vi "Display Info.vi"(7 "Layout ref":refnum<vi>, 8 "error in (no error)":errorcluster, 9 "Modify (F) /Add [T]":bool=TRUE, 10 "Names in use":string[](array[string])=["PB"], 11 "SRS_DS345 in":refnum<class "SRS_DS345.lvclass">=refnum) -> (0 "error out":errorcluster, 1 "Names in use out":string[](array[string]), 2 "Changes Made?":bool, 3 "SRS_DS345 out":refnum<class "SRS_DS345.lvclass">)   [LabVIEW 2013, in "SRS_DS345.lvclass"]
uses:
  SRS_DS345.lvclass
  ColumnVIs/SingleValCol/SingleValCol.lvclass
  TypeDefs/ColumnAppearCluster.ctl
  SRS_DS345.lvclass/SRS_DS345.ctl
  ColumnVIs/Column/Column.lvclass
panel:
  in  "Function Type Column Appearance":T1={"Column Name"="Func Type", "Width"=30, "Bkgd"=[16448250], "Text"=[0]}
  in  "Offset Column Appearance":T1={"Column Name"="Offset", "Width"=30, "Bkgd"=[16448250], "Text"=[0]}
  in  "Amplitude Column Apperance":T1={"Column Name"="Amplitude", "Width"=30, "Bkgd"=[16448250], "Text"=[0]}
  in  "Freq Column Appearance":T1={"Column Name"="Frequency", "Width"=30, "Bkgd"=[16448250], "Text"=[0]}
  in  "Cancel":bool
  in  "Done":bool
  in  "Hardware Settings":T2={"PB Trigger Line"=65535, "Serial Port"=""}
  in  "Device Description":string
  in  "Name":string
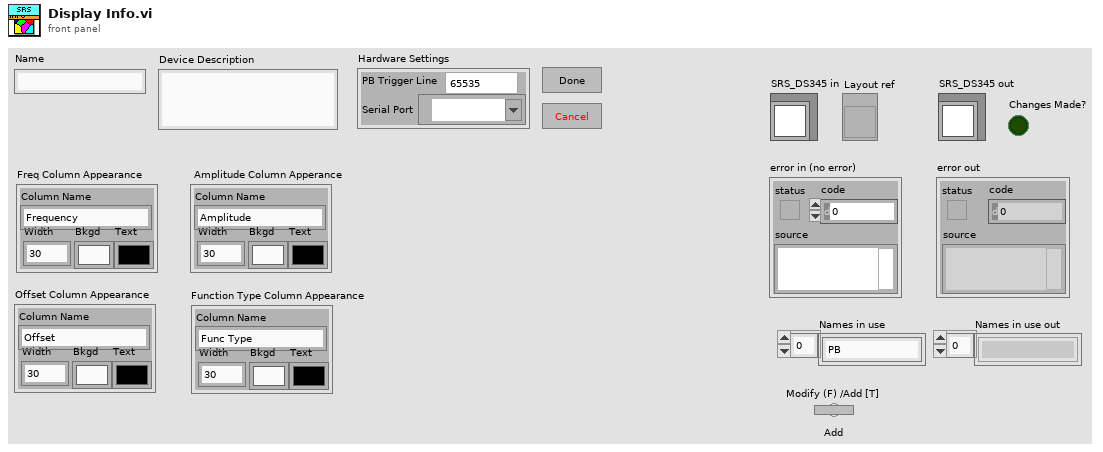
[diagram p1: front panel]
types:
  T1 = typedef "ColumnAppearCluster.ctl" = cluster{"Column Name":string, "Width":u32, "Bkgd":u32[], "Text":u32[]}
  T2 = cluster{"PB Trigger Line":u16, "Serial Port":refnum<visa-resource-name>}
  T3 = cluster{u16, "Serial Port":refnum<visa-resource-name>}
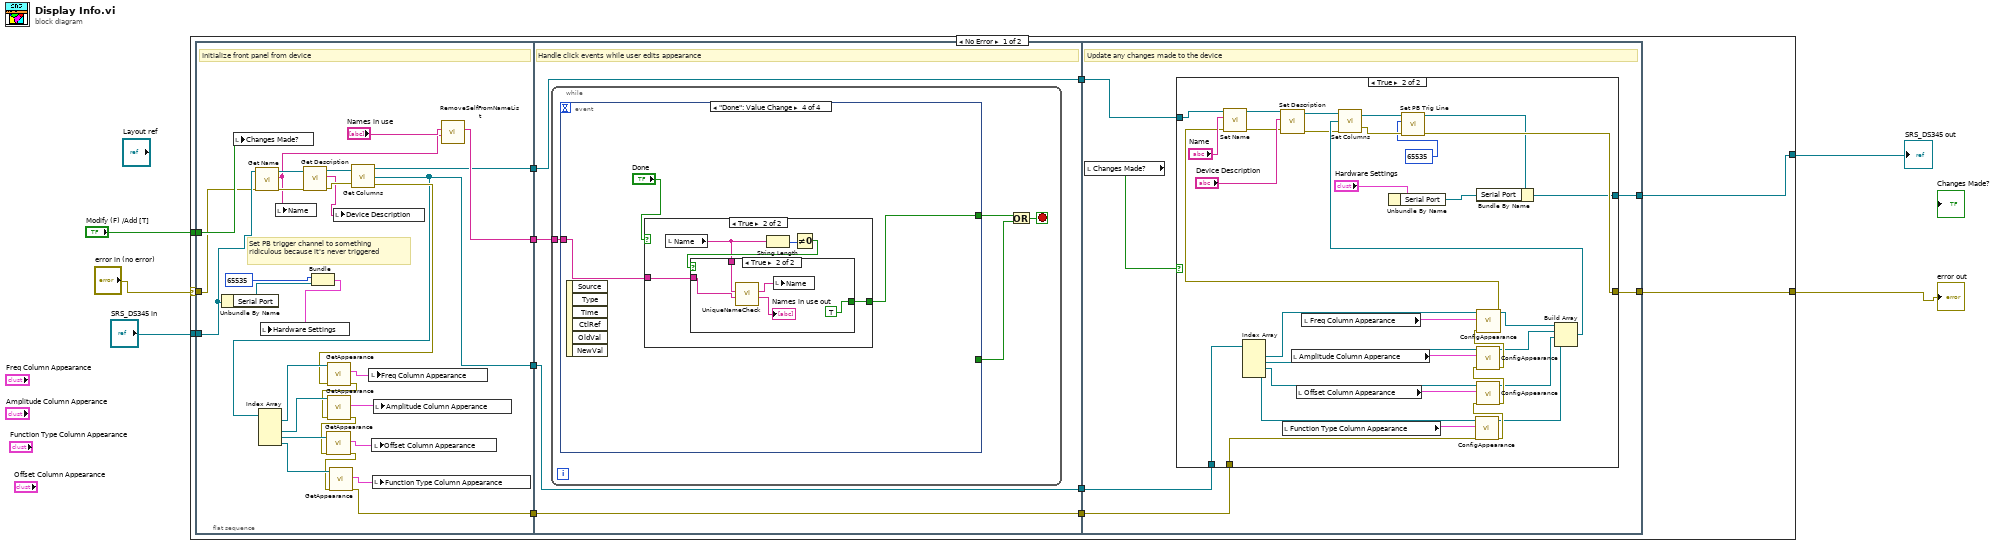
[diagram p0: block diagram]
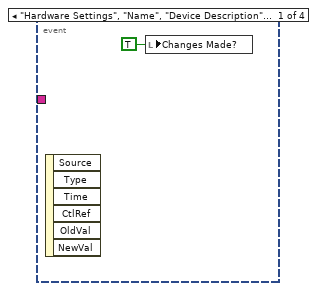
[diagram p2: hidden frame]
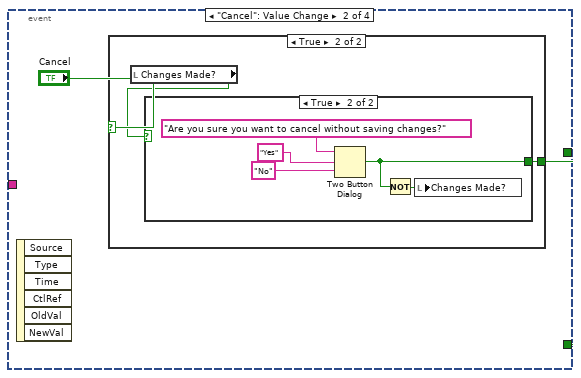
[diagram p3: hidden frame]
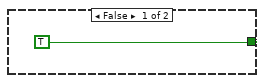
[diagram p5: hidden frame]
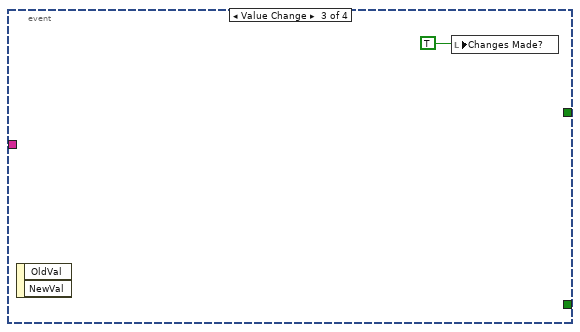
[diagram p6: hidden frame]
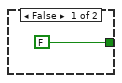
[diagram p7: hidden frame]
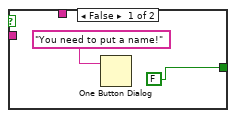
[diagram p8: hidden frame]
diagram:
  n1 = case shown="No Error" "error in (no error)" {
    selector: "error in (no error)" -> [w15 w127]
    tunnel: [w7 w127] -> w4
    tunnel: [w6 w126] -> w3
    tunnel: "SRS_DS345 in" -> [w16 w126]
    tunnel: "Modify (F) /Add [T]" -> [w17 _]
    frame No Error {
      n2 = flat-sequence {
        tunnel: w17 -> [w46]
        tunnel: w16 -> [w42]
        tunnel: w15 -> [w40]
        tunnel: [w21] -> w14
        tunnel: [w20] -> w13
        tunnel: [w19] -> w11
        tunnel: [w18] -> w9
        tunnel: w14 -> [w50]
        tunnel: w13 -> [w49]
        tunnel: [w49] -> w12
        tunnel: w11 -> [w48]
        tunnel: [w48] -> w10
        tunnel: w9 -> [w47]
        tunnel: [w47] -> w8
        tunnel: w12 -> [w89]
        tunnel: w10 -> [w88]
        tunnel: w8 -> [w87]
        tunnel: [w85] -> w7
        tunnel: [w84] -> w6
        frame #0 {
          # "Set PB trigger channel to something ridiculous because it's never triggered"
          # "Initialize front panel from device"
          n3 = Unbundle By Name(w42) -> ("Serial Port"=w44:refnum<visa-resource-name>)
          n4 = local write "Changes Made?"(w46) -> ()
          n5 = call-dynamic "Get Name.vi"("error in (no error)"=w40, "Device in"=w42) -> ("error out"=w39:errorcluster, "Name"=w35:string, "Device out"=w41:refnum<class "SRS_DS345.lvclass">)  [unwired: 7 in]
          n6 = local write "Name"(w35) -> ()
          n7 = call-dynamic "Get Description.vi"("error in (no error)"=w39, "Device in"=w41) -> ("error out"=w37:errorcluster, "Device Description"=w34:string, "Device out"=w38:refnum<class "SRS_DS345.lvclass">)  [unwired: 7 in]
          n8 = Bundle(u16 65535, "Serial Port"=w44) -> (w43:T3)  [unwired: 1 in]
          n9 = local write "Hardware Settings"(w43) -> ()
          n10 = local write "Device Description"(w34) -> ()
          n11 = call-dynamic "Get Columns.vi"("Device in"=w38, "error in (no error)"=w37) -> ("Device out"=w20:refnum<class "SRS_DS345.lvclass">, "Columns"=w19:refnum<class "Column.lvclass">[], "error out"=w29:errorcluster)
          n12 = Index Array(array=w19) -> (element #1=w33:refnum<class "Column.lvclass">, element #2=w32:refnum<class "Column.lvclass">, element #3=w31:refnum<class "Column.lvclass">, element #4=w30:refnum<class "Column.lvclass">)  [unwired: 4 in]
          n13 = call "GetAppearance.vi"("error in (no error)"=w29, "Column in"=w33) -> ("error out"=w28:errorcluster, "Column Appearance"=w25:T1)  [unwired: 7 in, 1 out]
          n14 = call "GetAppearance.vi"("error in (no error)"=w28, "Column in"=w32) -> ("error out"=w27:errorcluster, "Column Appearance"=w24:T1)  [unwired: 7 in, 1 out]
          n15 = call "GetAppearance.vi"("error in (no error)"=w27, "Column in"=w31) -> ("error out"=w26:errorcluster, "Column Appearance"=w23:T1)  [unwired: 7 in, 1 out]
          n16 = call "GetAppearance.vi"("error in (no error)"=w26, "Column in"=w30) -> ("error out"=w18:errorcluster, "Column Appearance"=w22:T1)  [unwired: 7 in, 1 out]
          n17 = local write "Freq Column Appearance"(w25) -> ()
          n18 = local write "Offset Column Appearance"(w23) -> ()
          n19 = local write "Function Type Column Appearance"(w22) -> ()
          n20 = local write "Amplitude Column Apperance"(w24) -> ()
          n21 = call "RemoveSelfFromNameList.vi"("self Name"=w35, "Names in use"="Names in use") -> ("Reserved Names"=w21:string[])  [unwired: 9 in]
        }
        frame #1 {
          # "Handle click events while user edits appearance"
          n22 = while {
            tunnel: w50 -> [w51]
            stop <- w54 stop-if-true
            n23 = event shown="[3] \"Done\": Value Change" {
              selector: _ -> [_ _ _ _]
              dyn-events: _ -> [_ _ _ _]
              timeout: _ -> [_ _ _ _]
              tunnel: [_ w57 _ _] -> w53
              tunnel: [_ _ _ w70] -> w52
              tunnel: w51 -> [_ _ _ w68]
              event "Hardware Settings", "Name", "Device Description": Value Change {
                n24 = event-data() -> ()  [unwired: 1 in, 6 out]
                n25 = local write "Changes Made?"(TRUE ("Changes Made?")) -> ()
              }
              event "Cancel": Value Change {
                n26 = event-data() -> ()  [unwired: 1 in, 6 out]
                n27 = case shown="True" "Cancel" {
                  selector: "Cancel" -> [w58 _]
                  tunnel: [w58 w60] -> w57
                  frame False {
                  }
                  frame True {
                    n28 = local read "Changes Made?"() -> (w59:bool)
                    n29 = case shown="True" w59 {
                      tunnel: [TRUE w63] -> w60
                      frame False {
                      }
                      frame True {
                        n30 = Two Button Dialog(message="Are you sure you want to cancel without saving changes?", 1:"No", 2:"Yes") -> (T button?=w63:bool)
                        n31 = Not(x=w63) -> (.not. x?=w62:bool)
                        n32 = local write "Changes Made?"(w62) -> ()
                      }
                    }
                  }
                }
              }
              event Value Change {
                n33 = event-data() -> ()  [unwired: 1 in, 2 out]
                n34 = local write "Changes Made?"(TRUE) -> ()
              }
              event "Done": Value Change {
                n35 = event-data() -> ()  [unwired: 1 in, 6 out]
                n36 = case shown="True" "Done" {
                  tunnel: [FALSE w74] -> w70
                  tunnel: w68 -> [_ w73]
                  frame False {
                  }
                  frame True {
                    n37 = local read "Name"() -> (w72:string)
                    n38 = String Length(string=w72) -> (length=w76:i32)
                    n39 = Not Equal To 0?(x=w76) -> (x != 0?=w75:bool)
                    n40 = case shown="True" w75 {
                      tunnel: [FALSE TRUE] -> w74
                      tunnel: w73 -> [_ w82]
                      tunnel: w72 -> [_ w81]
                      frame False {
                        n41 = One Button Dialog(message="You need to put a name!") -> ()  [unwired: 1 in, 1 out]
                      }
                      frame True {
                        n42 = call "UniqueNameCheck.vi"("Names in use"=w82, "Device Name"=w81) -> ("Names in use out"=→"Names in use out":string[], "Unique name"=w80:string)  [unwired: 8 in]
                        n43 = local write "Name"(w80) -> ()
                      }
                    }
                  }
                }
              }
            }
            n44 = Or(x=w52, y=w53) -> (x .or. y?=w54:bool)
          }
        }
        frame #2 {
          # "Update any changes made to the device"
          n45 = local read "Changes Made?"() -> (w86:bool)
          n46 = case shown="True" w86 {
            tunnel: w89 -> [w91 w125]
            tunnel: w88 -> [_ w120]
            tunnel: w87 -> [w90 w115]
            tunnel: [w90 w96] -> w85
            tunnel: [w91 w93] -> w84
            frame False {
            }
            frame True {
              n47 = Index Array(array=w120) -> (element #1=w119:refnum<class "Column.lvclass">, element #2=w118:refnum<class "Column.lvclass">, element #3=w117:refnum<class "Column.lvclass">, element #4=w116:refnum<class "Column.lvclass">)  [unwired: 4 in]
              n48 = local read "Function Type Column Appearance"() -> (w106:T1)
              n49 = local read "Amplitude Column Apperance"() -> (w108:T1)
              n50 = local read "Offset Column Appearance"() -> (w107:T1)
              n51 = local read "Freq Column Appearance"() -> (w109:T1)
              n52 = Unbundle By Name("Hardware Settings") -> ("Serial Port"=w94:refnum<visa-resource-name>)
              n53 = call "ConfigAppearance.vi"("error in (no error)"=w115, "Column Appearance"=w106, "Column in"=w116) -> ("error out"=w114:errorcluster, "Column out"=w102:refnum<class "Column.lvclass">)  [unwired: 7 in]
              n54 = call "ConfigAppearance.vi"("error in (no error)"=w114, "Column Appearance"=w107, "Column in"=w117) -> ("error out"=w113:errorcluster, "Column out"=w103:refnum<class "Column.lvclass">)  [unwired: 7 in]
              n55 = call "ConfigAppearance.vi"("error in (no error)"=w113, "Column Appearance"=w108, "Column in"=w118) -> ("error out"=w112:errorcluster, "Column out"=w104:refnum<class "Column.lvclass">)  [unwired: 7 in]
              n56 = call "ConfigAppearance.vi"("error in (no error)"=w112, "Column Appearance"=w109, "Column in"=w119) -> ("error out"=w111:errorcluster, "Column out"=w105:refnum<class "Column.lvclass">)  [unwired: 7 in]
              n57 = call-dynamic "Set Name.vi"("error in (no error)"=w111, "Name"="Name", "Device in"=w125) -> ("error out"=w110:errorcluster, "Device out"=w123:refnum<class "SRS_DS345.lvclass">)  [unwired: 7 in]
              n58 = call-dynamic "Set Description.vi"("error in (no error)"=w110, "Device Description"="Device Description", "Device in"=w123) -> ("error out"=w99:errorcluster, "Device out"=w100:refnum<class "SRS_DS345.lvclass">)  [unwired: 7 in]
              n59 = Build Array(w105, w104, w103, w102) -> (w101:refnum<class "Column.lvclass">[])
              n60 = call-dynamic "Set Columns.vi"("error in (no error)"=w99, "Columns"=w101, "Device in"=w100) -> ("error out"=w97:errorcluster, "Device out"=w98:refnum<class "SRS_DS345.lvclass">)  [unwired: 1 in]
              n61 = call-dynamic "Set PB Trig Line.vi"("error in (no error)"=w97, "PB Trigger Line"=u16 65535, "Device in"=w98) -> ("error out"=w96:errorcluster, "Device out"=w95:refnum<class "SRS_DS345.lvclass">)  [unwired: 7 in]
              n62 = Bundle By Name(cluster=w95, "Serial Port"=w94) -> (w93:refnum<class "SRS_DS345.lvclass">)
            }
          }
        }
      }
    }
    frame Error {
    }
  }
  "error out" <- w4
  "SRS_DS345 out" <- w3
